vi "Excel_to_graph_2.vi"() -> ()   [LabVIEW 2016]
uses:
  <vilib>/addons/_office/excel.llb/Excel Get Data ([str]).vi
  <vilib>/Utility/NIReport.llb/NI_report.lvclass
  <vilib>/addons/_office/NI_ReportGenerationToolkit.lvlib
  <vilib>/Utility/NIReport.llb/Excel/NI_Excel.lvclass
panel:
  in  "data 2":string[][](array[string])
  in  "Excel?":bool=TRUE
  out "回放秒數":u32
  out "?":i32[][](graph)
  in  "File name":path
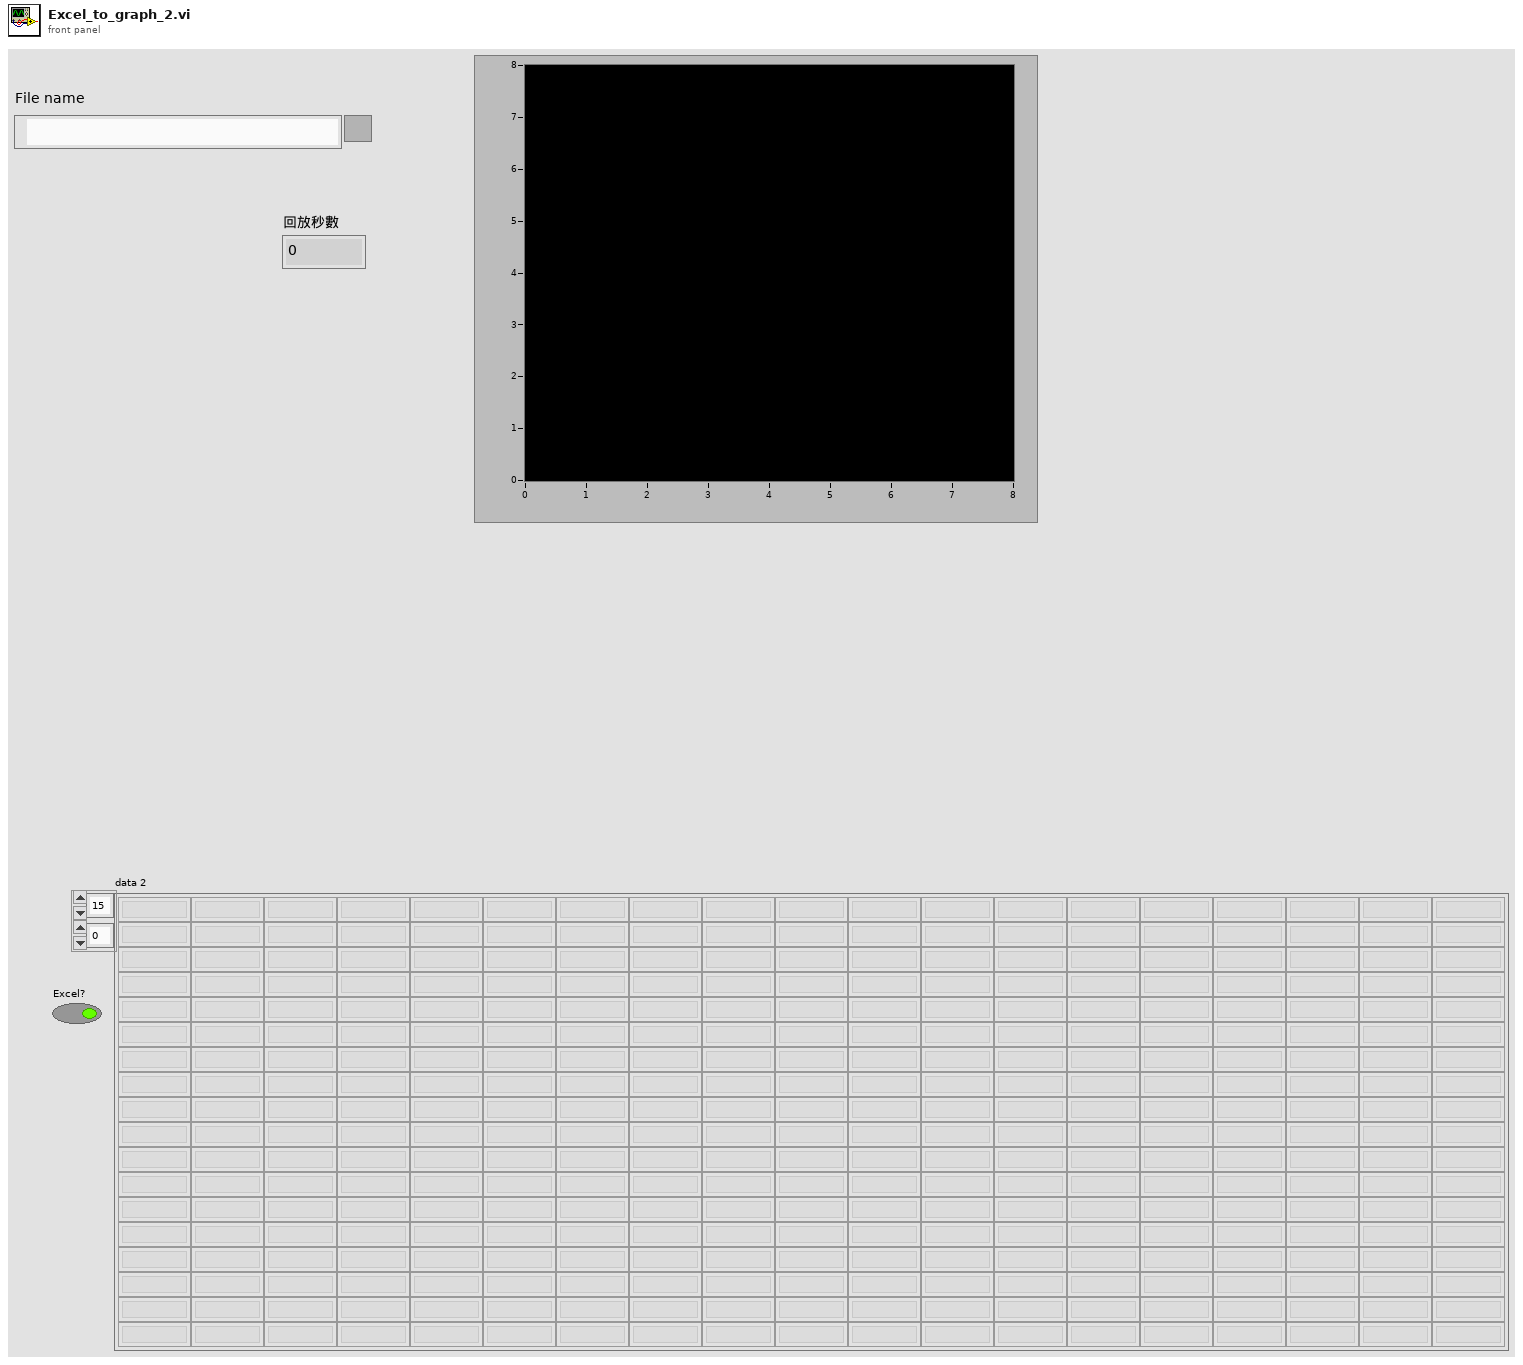
[diagram p1: front panel]
types:
  T1 = enum16{"maximized", "minimized", "normal", "no change"}
  T2 = enum16{"Standard Report", "HTML", "Word", "Excel"}
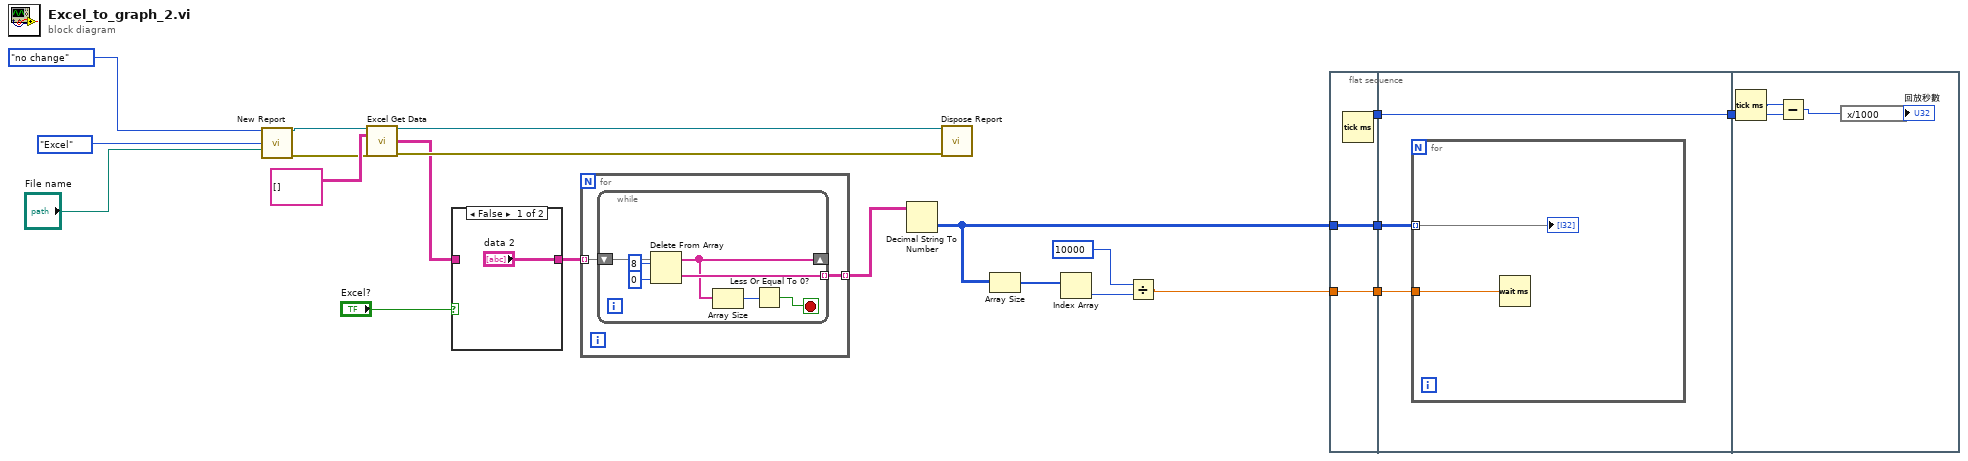
[diagram p0: block diagram]
diagram:
  n1 = call <vilib>:"New Report.vi"("window state (normal)"=T1."no change", "report type"=T2."Excel", "template (empty)"="File name") -> ("report out"=w18:refnum<class "NI_report.lvclass">, "error out"=w8:errorcluster)  [unwired: 11 in]
  n2 = call-poly <vilib>:"Excel Get Data.vi"("report in"=w18, "data type"=string[][] [], "error in (no error)"=w8) -> ("report out"=w16:refnum<class "NI_report.lvclass">, "data"=w2:string[][], "error out"=w15:errorcluster)  [unwired: 10 in]
  n3 = case shown="False" "Excel?" {
    tunnel: w2 -> [_ w23]
    tunnel: ["data 2" w23] -> w1
    frame False {
    }
    frame True {
    }
  }
  n4 = for {
    tunnel: w1 -> [w25] mode=indexing
    tunnel: [w24] -> w9 mode=indexing
    n5 = while {
      shift-right: [w28] -> _
      shift-left: w25 -> [w32]
      tunnel: [w29] -> w24 mode=indexing
      stop <- w26 stop-if-true
      n6 = Delete From Array(array=w32, length=8, index=0) -> (deleted portion=w29:string[], array with subset deleted=w28:string[])
      n7 = Array Size(array=w28) -> (size(s)=w27:i32)
      n8 = Less Or Equal To 0?(x=w27) -> (x <= 0?=w26:bool)
    }
  }
  n9 = Decimal String To Number(string=w9) -> (number=w10:i32[][][])  [unwired: 2 in, 1 out]
  n10 = call-dynamic "Dispose Report.vi"("report in"=w16, "error in (no error)"=w15) -> ()  [unwired: 13 in, 1 out]
  n11 = Array Size(array=w10) -> (size(s)=w14:i32[])
  n12 = Index Array(array=w14) -> (element=w13:i32)  [unwired: 1 in]
  n13 = Divide(x=10000, y=w13) -> (x/y=w11:dbl)
  n14 = flat-sequence {
    tunnel: w10 -> [w34]
    tunnel: w11 -> [w35]
    tunnel: [w35] -> w7
    tunnel: [w34] -> w6
    tunnel: [w33] -> w5
    tunnel: w7 -> [w38]
    tunnel: w6 -> [w37]
    tunnel: w5 -> [w36]
    tunnel: [w36] -> w4
    tunnel: w4 -> [w43]
    frame #0 {
      n15 = Tick Count (ms)() -> (millisecond timer value=w33:u32)
    }
    frame #1 {
      n16 = for {
        tunnel: w38 -> [w40]
        tunnel: w37 -> [w39] mode=indexing
        n17 = Wait (ms)(milliseconds to wait=w40) -> ()  [unwired: 1 out]
        "?" <- w39
      }
    }
    frame #2 {
      n18 = Tick Count (ms)() -> (millisecond timer value=w44:u32)
      n19 = Subtract(x=w44, y=w43) -> (x-y=w42:u32)
      n20 = expression code="x/1000"(w42) -> (→"回放秒數":u32)
    }
  }
